vi "Get Input Channel.vi"(0 "Input Channels[]":refnum<class "Input Channels.lvclass">[](array[class]), 11 "error in (no error)":errorcluster) -> (3 "Scale Active?":bool, 4 "Input Channel Details[][]":string[][](array[string]), 6 "Channel Selection[]":i32[](array[numeric]), 8 "Active Channels[]":string[](array[string]), 10 "Select All":enum8{"False", "True", "Mixed"}(ring), 14 "Refresh (ms)":dbl, 15 "error out":errorcluster)   [LabVIEW 2020, in "Plugin.lvlib" / "Plugin_UI.lvclass"]
doc: "Reads all the input channel details required for updating the Configuration Interface."
uses:
  Plugin_UI.lvclass
  Channels/Input Channels/Input Channels.lvclass
  C:/SVN_LabSys/labsys_lvcode/LabSys_SourceCode/Plugin Template/Source/Code/Channels/Plugin_Channels.lvclass
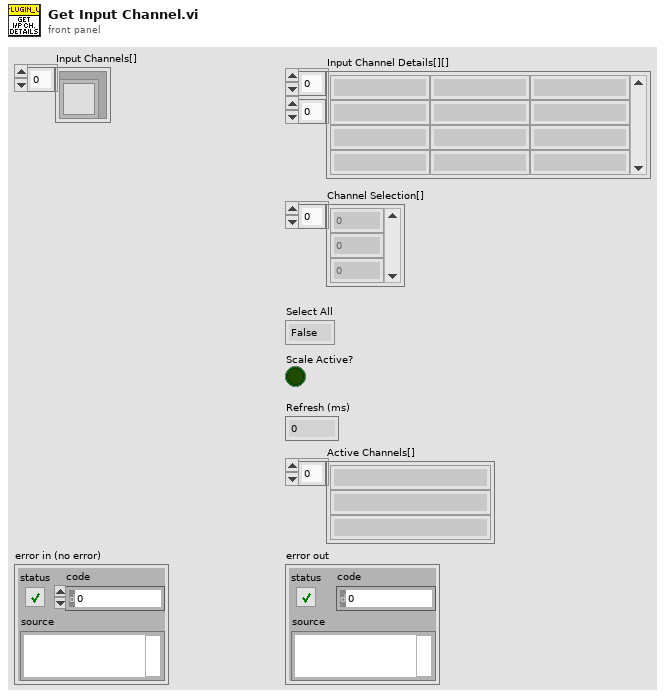
[diagram p1: front panel]
types:
  T1 = typedef "LabSys Framework.lvlibp/Configuration Storage.lvlib/Test Configuration.lvclass/Scaling Information.ctl" = cluster{"Active":bool, "Scaling Type":T2, "Output Minimum":dbl, "Output Maximum":dbl, "Raw Minimum":dbl, "Raw Maximum":dbl, "Output Unit":string, "Function":string, "Lookup Table":string}
  T2 = typedef "LabSys Framework.lvlibp/Configuration Storage.lvlib/Test Configuration.lvclass/Scaling Types.ctl" = enum8{"Linear", "Function", "Lookup Table"}
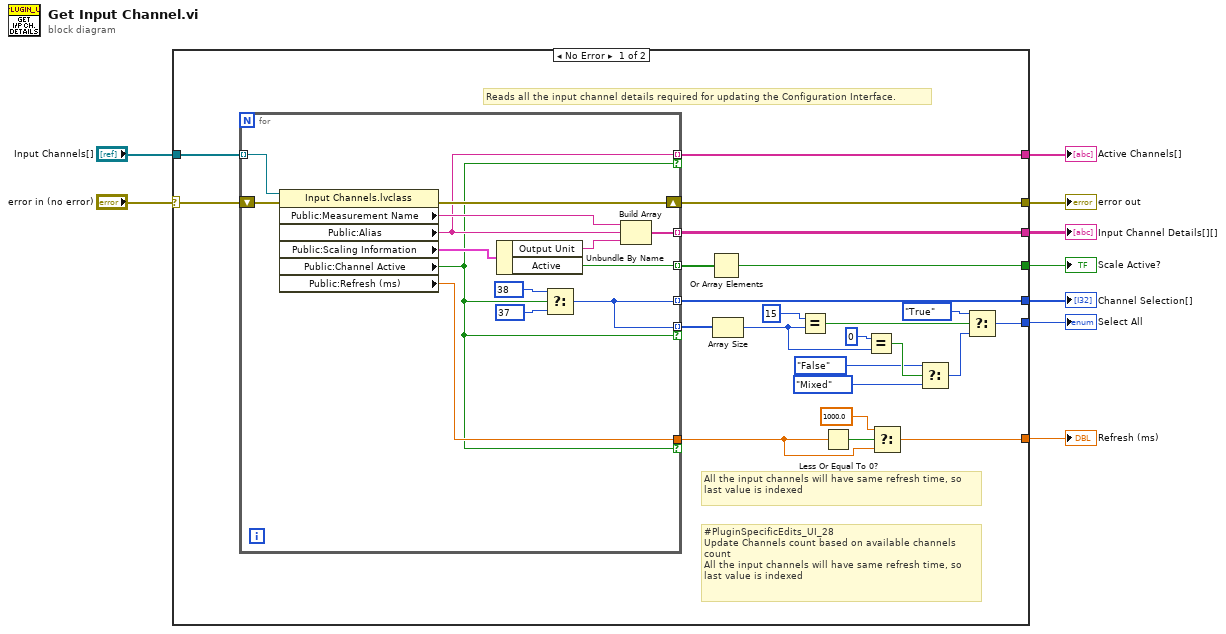
[diagram p0: block diagram]
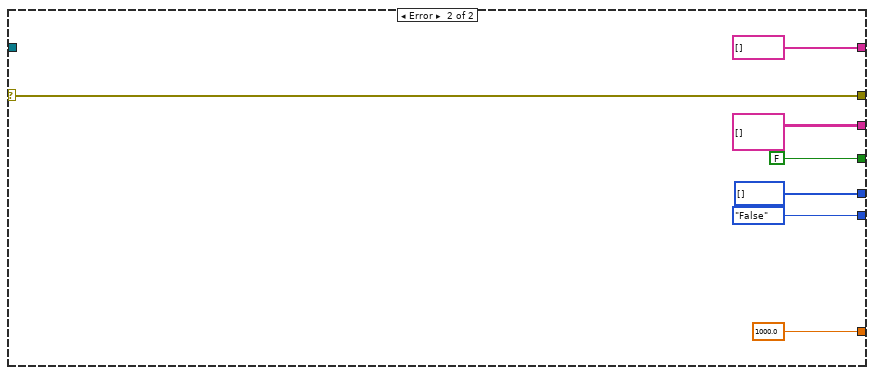
[diagram p2: hidden frame]
diagram:
  n1 = case shown="No Error" "error in (no error)" {
    selector: "error in (no error)" -> [w26 w53]
    tunnel: "Input Channels[]" -> [w32 _]
    tunnel: [w31 string[][] []] -> w8
    tunnel: [w30 i32[] []] -> w7
    tunnel: [w29 w53] -> w6
    tunnel: [w27 FALSE] -> w5
    tunnel: [w15 enum8{"False", "True", "Mixed"}."False" ("Select All")] -> w3
    tunnel: [w11 1000.0 ("Public:Refresh (ms)")] -> w2
    tunnel: [w10 string[] []] -> w1
    frame No Error {
      # "All the input channels will have same refresh time, so last value is indexed"
      # "Reads all the input channel details required for updating the Configuration Interface."
      # "#PluginSpecificEdits_UI_28\nUpdate Channels count based on available channels count\nAll the input channels will have same refresh time, so last value is indexed"
      n2 = for {
        tunnel: w32 -> [w45] mode=indexing
        shift-right: [w42] -> w29
        shift-left: w26 -> [w46]
        tunnel: [w41] -> w31 mode=indexing
        tunnel: [w36] -> w30 mode=indexing
        tunnel: [w38] -> w28 mode=indexing
        tunnel: [w36] -> w25 mode=indexing if=w33
        tunnel: [w35] -> w13 if=w33
        tunnel: [w34] -> w10 mode=indexing if=w33
        n3 = property class="Input Channels.lvclass"(reference=w45, error in=w46) -> (error out=w42:errorcluster, "Public:Measurement Name"=w44:string, "Public:Alias"=w34:string, "Public:Scaling Information"=w37:T1, "Public:Channel Active"=w33:bool, "Public:Refresh (ms)"=w35:dbl)  [unwired: 1 out]
        n4 = Unbundle By Name(w37) -> ("Output Unit"=w43:string, "Active"=w38:bool)
        n5 = Select(t=38, s=w33, f=37) -> (s? t:f=w36:i32)
        n6 = Build Array(w44, w34, w43) -> (w41:string[])
      }
      n7 = Or Array Elements(Boolean array=w28) -> (logical OR=w27:bool)
      n8 = Array Size(array=w25) -> (size(s)=w16:i32)
      n9 = Equal?(x=15, y=w16) -> (x = y?=w24:bool)
      n10 = Less Or Equal To 0?(x=w13) -> (x <= 0?=w14:bool)
      n11 = Equal?(x=0, y=w16) -> (x = y?=w19:bool)
      n12 = Select(t=1000.0, s=w14, f=w13) -> (s? t:f=w11:dbl)
      n13 = Select(t=enum8{"False", "True", "Mixed"}."False" ("Select All"), s=w19, f=enum8{"False", "True", "Mixed"}."Mixed" ("Select All")) -> (s? t:f=w23:enum8{"False", "True", "Mixed"})
      n14 = Select(t=enum8{"False", "True", "Mixed"}."True" ("Select All"), s=w24, f=w23) -> (s? t:f=w15:enum8{"False", "True", "Mixed"})
    }
    frame Error {
    }
  }
  "Input Channel Details[][]" <- w8
  "Channel Selection[]" <- w7
  "error out" <- w6
  "Scale Active?" <- w5
  "Select All" <- w3
  "Refresh (ms)" <- w2
  "Active Channels[]" <- w1
